vi "optagefrekvenssignal0.6.vi"() -> ()   [LabVIEW 2014]
uses:
  <vilib>/measure/maspectr.llb/FFT Power Spectrum and PSD for 1 Chan.vi
  <vilib>/measure/NI_MAPro.lvlib
panel:
  out "Resonansfrekvens":dbl[](array[numeric])
  out "Volumen(ml)":dbl[](array[numeric])
  in  "Tid":dbl
  out "Maks frekvens":dbl
  out "FFT af lydsignal":dbl[](graph)
  out "Lydsignal":waveform(dbl)(graph)
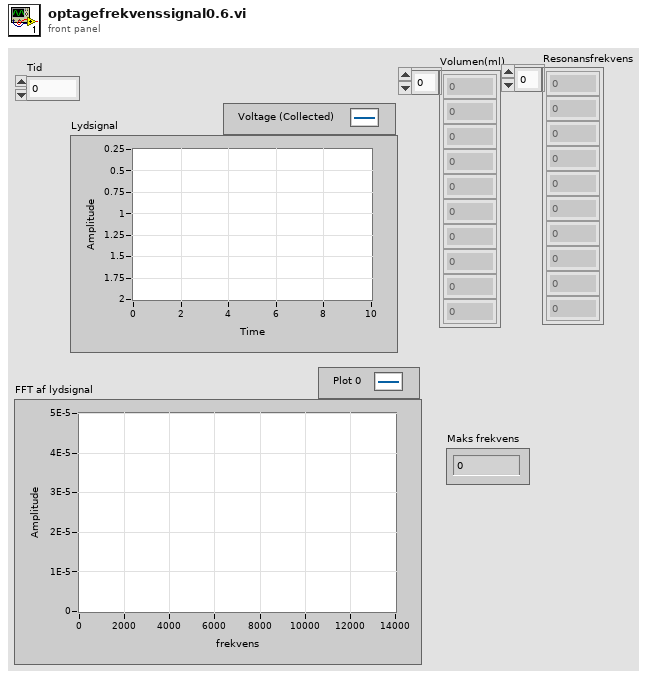
[diagram p1: front panel]
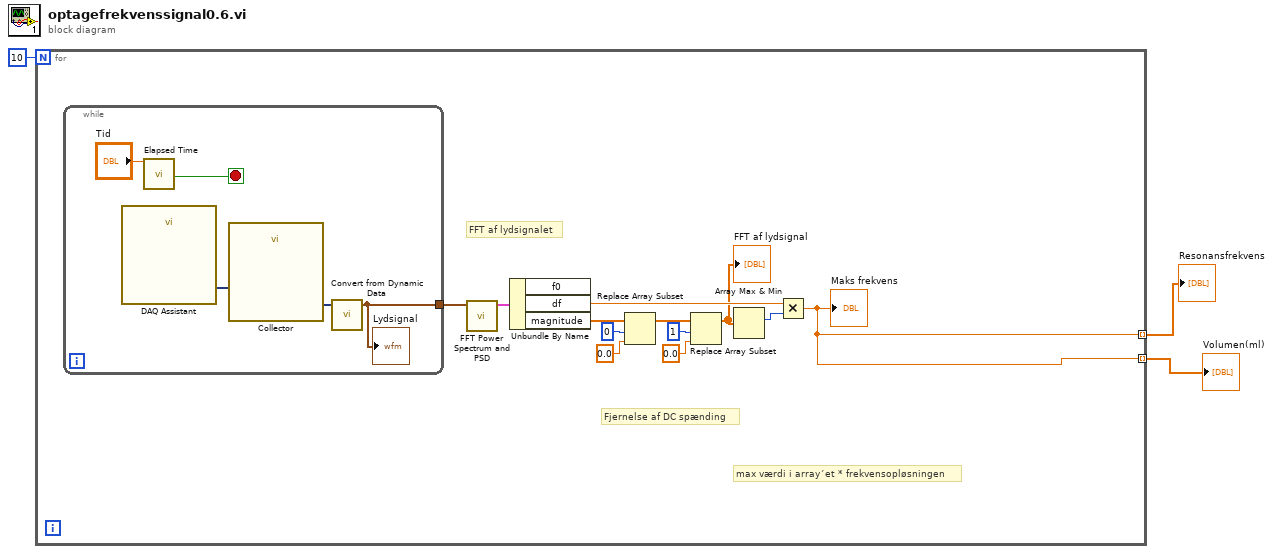
[diagram p0: block diagram]
diagram:
  n1 = for {
    N: 10 -> [_]
    tunnel: [w4] -> w2 mode=indexing
    tunnel: [w4] -> w1 mode=indexing
    # "max værdi i array´et * frekvensopløsningen"
    # "Fjernelse af DC spænding"
    # "FFT af lydsignalet"
    n2 = while {
      tunnel: [w20] -> w15
      stop <- w16 stop-if-true
      n3 = call "DAQ Assistant"() -> ("data"=w19:dynamicdata)  [unwired: 17 in, 2 out]
      n4 = call "Elapsed Time"("Time Target (s)"="Tid") -> ("Time has Elapsed"=w16:bool)  [unwired: 11 in, 7 out]
      n5 = call "Collector"("Signals"=w19) -> ("Collected Signals"=w18:dynamicdata)  [unwired: 9 in, 1 out]
      n6 = call "Convert from Dynamic Data"("Dynamic Data Type"=w18) -> ("Waveform"=w20:waveform(dbl))  [unwired: 3 in]
      "Lydsignal" <- w20
    }
    n7 = call-poly <vilib>:"FFT Power Spectrum and PSD.vi"("time signal"=w15) -> ("Power Spectrum / PSD"=w7:cluster{"f0":dbl, "df":dbl, "magnitude":dbl[]})  [unwired: 7 in, 3 out]
    n8 = Unbundle By Name(w7) -> ("df"=w8:dbl, "magnitude"=w6:dbl[])  [unwired: 1 out]
    n9 = Replace Array Subset(array=w6, new element=0.0 ("new element/subarray"), index=0) -> (w12:dbl[])
    n10 = Replace Array Subset(array=w12, new element=0.0 ("new element/subarray"), index=1) -> (w5:dbl[])
    "FFT af lydsignal" <- w5
    n11 = Array Max & Min(array=w5) -> (max index (indices)=w9:i32)  [unwired: 3 out]
    n12 = Multiply(x=w8, y=w9) -> (x*y=w4:dbl)
    "Maks frekvens" <- w4
  }
  "Volumen(ml)" <- w2
  "Resonansfrekvens" <- w1
